vi "VelocityProfile.vi"(0 "t":dbl, 1 "a1":dbl=10.0, 3 "a3":dbl=15.0, 5 "s":dbl, 7 "intervalo":dbl=0.016, 9 "v_est":dbl, 11 "v_max":dbl=3.0, 12 "v3":dbl, 13 "s3":dbl) -> (4 "Velocity":dbl, 6 "VelocityProfileState Out":T1, 8 "Velocities":dbl[](array[numeric]), 10 "Time":dbl[](array[numeric]))   [LabVIEW 2023]
uses:
  Controle/VelocityProfileState.ctl
panel:
  out "Amax":dbl=8.0
  in  "Reset":bool
  out "Velocity Profile":cluster{dbl[], dbl[]}(graph)
  in  "Tolerancia Vel":dbl=0.01
  in  "Tolerancia Pos":dbl=0.010000000000000004
  out "VelocityProfileState In":T1={"t0"=0.0, "t1"=0.0, "t2"=0.0, "t3"=0.0, "v0"=0.0, "v_max"=3.0, "v3"=0.0, "v2"=0.0, "v1"=0.0, "perfil"=enum."Triangular", "regiao"=0, "s0"=0.0, "s1"=0.0, "s2"=0.0, "v"=0.0, "t"=0.0, "a1"=10.0, "s3"=0.0, "Reset"=FALSE, "s"=0.0, "a3"=15.0, "Ré"=FALSE, "Impossível"=FALSE, "intervalo"=0.0}
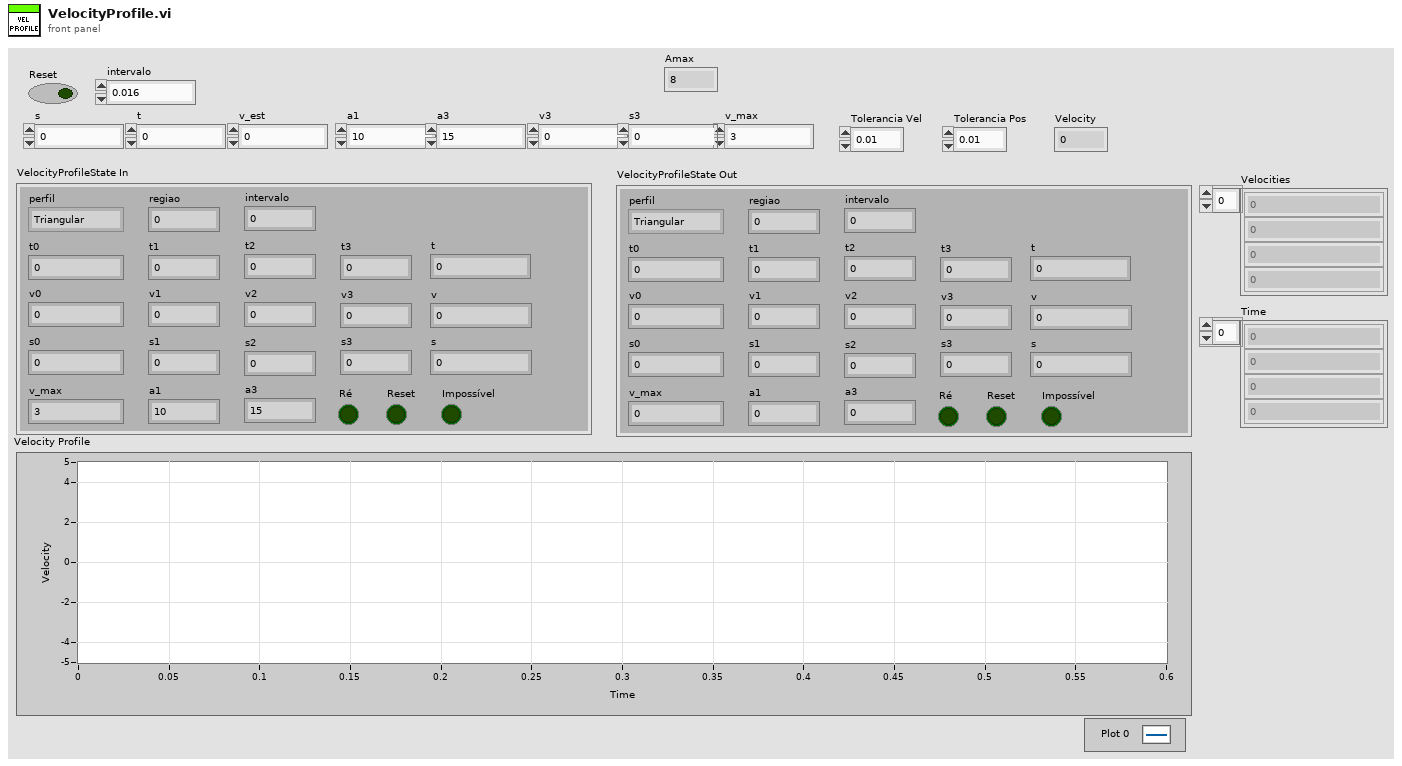
[diagram p1: front panel]
types:
  T1 = typedef "VelocityProfileState.ctl" = cluster{"t0":dbl, "t1":dbl, "t2":dbl, "t3":dbl, "v0":dbl, "v_max":dbl, "v3":dbl, "v2":dbl, "v1":dbl, "perfil":enum16{"Triangular", "Trapezoidal"}, "regiao":i32, "s0":dbl, "s1":dbl, "s2":dbl, "v":dbl, "t":dbl, "a1":dbl, "s3":dbl, "Reset":bool, "s":dbl, "a3":dbl, "Ré":bool, "Impossível":bool, "intervalo":dbl}
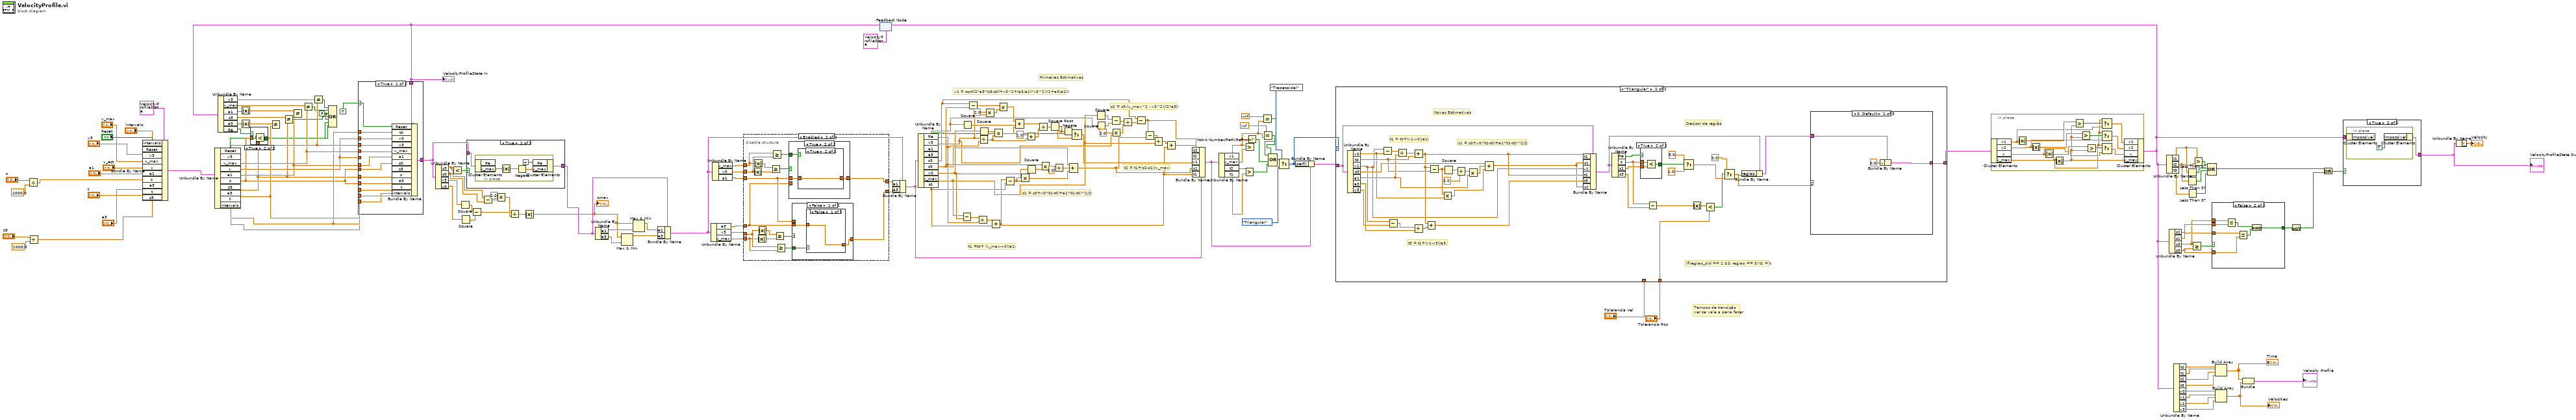
[diagram p0: block diagram]
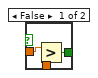
[diagram p2: hidden frame]
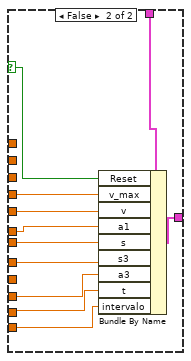
[diagram p3: hidden frame]
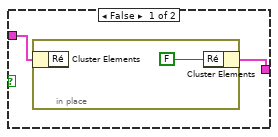
[diagram p4: hidden frame]
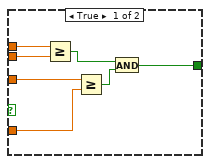
[diagram p5: hidden frame]
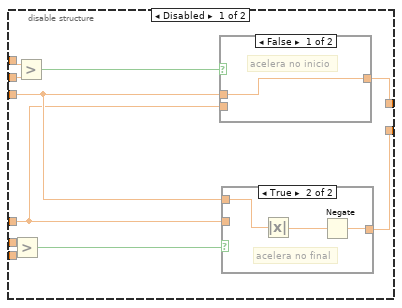
[diagram p6: hidden frame]
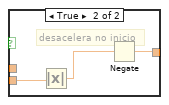
[diagram p8: hidden frame]
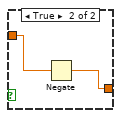
[diagram p9: hidden frame]
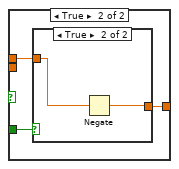
[diagram p10: hidden frame]
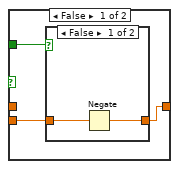
[diagram p12: hidden frame]
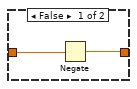
[diagram p14: hidden frame]
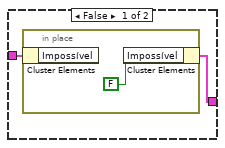
[diagram p15: hidden frame]
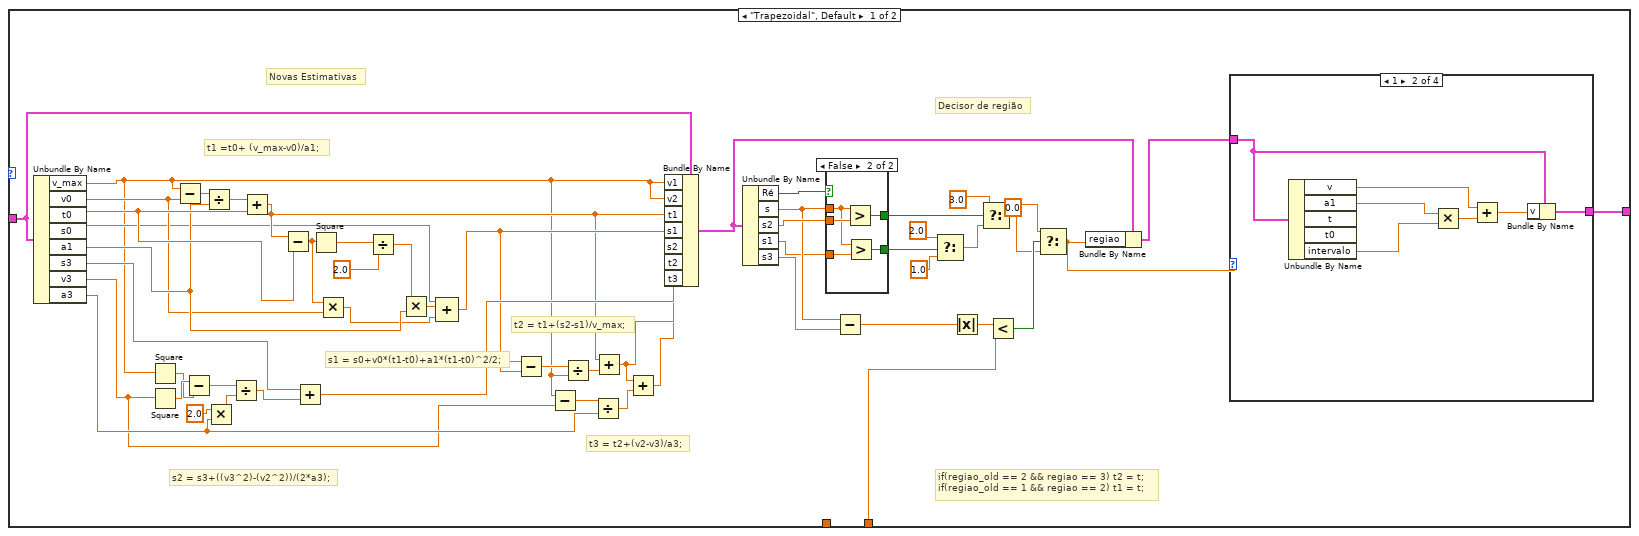
[diagram p16: hidden frame]
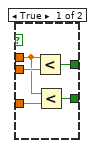
[diagram p17: hidden frame]
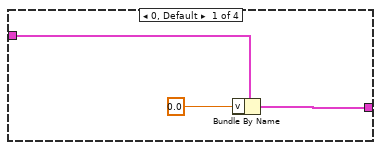
[diagram p18: hidden frame]
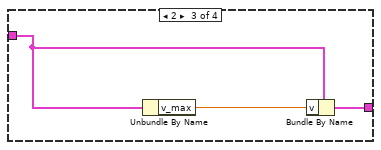
[diagram p19: hidden frame]
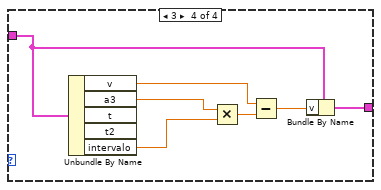
[diagram p20: hidden frame]
diagram:
  w40 = FALSE ("value")
  # "Tempos de transição\nver se vale a pena fazer"
  # "Primeiras Estimativas"
  # "t2 = t1+(s2-s1)/v_max;"
  # "s2 = s3-(v_max^2 - v3^2)/(2*a3);"
  # "s1 = s0+v0*(t1-t0)+a1*(t1-t0)^2/2;"
  # "t1 =t0+ (v_max-v0)/a1;"
  # "v1 = sqrt((2*a3*(s3-s0)+v3^2+(a3/a1)*v0^2)/(1+a3/a1));"
  n1 = Divide(x="s", y=1000.0) -> (x/y=w149:dbl)
  n2 = Divide(x="s3", y=1000.0) -> (x/y=w150:dbl)
  n3 = Bundle By Name(cluster=T1 {"t0"=0.0, "t1"=0.0, "t2"=0.0, "t3"=0.0, "v0"=0.0, "v_max"=0.0, "v3"=0.0, "v2"=0.0, "v1"=0.0, "perfil"=enum."Triangular", "regiao"=0, "s0"=0.0, "s1"=0.0, "s2"=0.0, "v"=0.0, "t"=0.0, "a1"=0.0, "s3"=0.0, "Reset"=FALSE, "s"=0.0, "a3"=0.0, "Ré"=FALSE, "Impossível"=FALSE, "intervalo"=0.0} ("VelocityProfileState In"), "intervalo"="intervalo", "Reset"="Reset", "v3"="v3", "v_max"="v_max", "v"="v_est", "a1"="a1", "s"=w149, "a3"="a3", "t"="t", "s3"=w150) -> (w155:T1)
  n4 = Unbundle By Name(w155) -> ("Reset"=w42:bool, "v3"=w128:dbl, "v_max"=w126:dbl, "v"=w56:dbl, "a1"=w55:dbl, "s"=w44:dbl, "s3"=w43:dbl, "a3"=w60:dbl, "t"=w57:dbl, "intervalo"=w35:dbl)
  n5 = feedback #1(T1 {"t0"=0.0, "t1"=0.0, "t2"=0.0, "t3"=0.0, "v0"=0.0, "v_max"=0.0, "v3"=0.0, "v2"=0.0, "v1"=0.0, "perfil"=enum."Triangular", "regiao"=0, "s0"=0.0, "s1"=0.0, "s2"=0.0, "v"=0.0, "t"=0.0, "a1"=0.0, "s3"=0.0, "Reset"=FALSE, "s"=0.0, "a3"=0.0, "Ré"=FALSE, "Impossível"=FALSE, "intervalo"=0.0} ("VelocityProfileState In")) -> (w25:T1)
  "VelocityProfileState In" <- w25
  n6 = Unbundle By Name(w25) -> ("v3"=w129:dbl, "v_max"=w127:dbl, "a1"=w48:dbl, "s3"=w125:dbl, "a3"=w47:dbl, "Ré"=w45:bool)
  n7 = Absolute Value(x=w48) -> (abs(x)=w49:dbl)
  n8 = Absolute Value(x=w47) -> (abs(x)=w46:dbl)
  n9 = case shown="True" w45 {
    tunnel: w44 -> [w167 w170]
    tunnel: w43 -> [w166 w169]
    tunnel: [w165 w168] -> w41
    frame False {
      n10 = Greater?(x=w167, y=w166) -> (0:w165:bool)
    }
    frame True {
      n11 = Less?(x=w170, y=w169) -> (x < y?=w168:bool)
    }
  }
  n12 = Not Equal?(x=w46, y=w60) -> ()  [unwired: 1 out]
  n13 = Not Equal?(x=w125, y=w43) -> (x != y?=w122:bool)
  n14 = Not Equal?(x=w49, y=w55) -> ()  [unwired: 1 out]
  n15 = Not Equal?(x=w127, y=w126) -> (x != y?=w123:bool)
  n16 = Not Equal?(x=w129, y=w128) -> (x != y?=w124:bool)
  n17 = Compound Arithmetic op=OR(w124, w123, w40, w122, w40, w41, w42) -> ()  [unwired: 1 out]
  n18 = case shown="True" TRUE {
    selector: TRUE -> [w178 w191]
    tunnel: w57 -> [w184 _]
    tunnel: w56 -> [w183 _]
    tunnel: w128 -> [w182 _]
    tunnel: w126 -> [w181 w195]
    tunnel: w56 -> [_ w194]
    tunnel: [w180 w193] -> w146
    tunnel: w25 -> [w179 w192]
    tunnel: w60 -> [w177 w190]
    tunnel: w57 -> [w176 w189]
    tunnel: w44 -> [w175 _]
    tunnel: w55 -> [w171 w188]
    tunnel: w44 -> [w174 w187]
    tunnel: w43 -> [w173 w186]
    tunnel: w35 -> [w172 w185]
    frame True {
      n19 = Bundle By Name(cluster=w179, "Reset"=w178, "t0"=w184, "v0"=w183, "v3"=w182, "v_max"=w181, "a1"=w171, "s0"=w174, "s3"=w173, "s"=w175, "a3"=w177, "t"=w176, "intervalo"=w172) -> (w180:T1)
    }
    frame False {
      n20 = Bundle By Name(cluster=w192, "Reset"=w191, "v_max"=w195, "v"=w194, "a1"=w188, "s"=w187, "s3"=w186, "a3"=w190, "t"=w189, "intervalo"=w185) -> (w193:T1)
    }
  }
  n21 = Unbundle By Name(w146) -> ("s3"=w10:dbl, "s0"=w9:dbl, "v3"=w14:dbl, "v0"=w13:dbl)
  n22 = Less?(x=w10, y=w9) -> (x < y?=w59:bool)
  n23 = Square(x=w14) -> (x^2=w12:dbl)
  n24 = Square(x=w13) -> (x^2=w11:dbl)
  n25 = case shown="True" w59 {
    tunnel: w146 -> [w197 w200]
    tunnel: [w196 w199] -> w21
    frame False {
      n26 = in-place {
        n27 = in-place-cluster #2(w197) -> ()  [unwired: 1 out]
        n28 = in-place-cluster #2("Ré"=FALSE) -> (w196:T1)
      }
    }
    frame True {
      n29 = in-place {
        n30 = in-place-cluster #3(w200) -> ("v_max"=w204:dbl)  [unwired: 1 out]
        n31 = Absolute Value(x=w204) -> (abs(x)=w203:dbl)
        n32 = Negate(x=w203) -> (-x=w202:dbl)
        n33 = in-place-cluster #3("Ré"=TRUE, "v_max"=w202) -> (w199:T1)
      }
    }
  }
  n34 = Subtract(x=w12, y=w11) -> (x-y=w6:dbl)
  n35 = Subtract(x=w10, y=w9) -> (x-y=w8:dbl)
  n36 = Multiply(x=2.0, y=w8) -> (x*y=w5:dbl)
  n37 = Divide(x=w6, y=w5) -> (x/y=w4:dbl)
  n38 = Absolute Value(x=w4) -> (abs(x)=w3:dbl)
  "Amax" <- w3
  n39 = Unbundle By Name(w21) -> ("a1"=w20:dbl, "a3"=w19:dbl)
  n40 = Max & Min(x=w3, y=w19) -> (max(x,y)=w1:dbl)  [unwired: 1 out]
  n41 = Max & Min(x=w3, y=w20) -> (max(x,y)=w2:dbl)  [unwired: 1 out]
  n42 = Bundle By Name(cluster=w21, "a1"=w2, "a3"=w1) -> (w22:T1)
  n43 = Unbundle By Name(w22) -> ("a3"=w61:dbl, "v3"=w106:dbl, "v_max"=w107:dbl)
  n44 = Unbundle By Name(w22) -> ("v_max"=w145:dbl, "v0"=w144:dbl, "a1"=w62:dbl)
  n45 = disable-structure shown="Enabled" {
    disable-tunnel: w145 -> [w214 w234]
    disable-tunnel: w144 -> [w213 w233]
    disable-tunnel: w107 -> [w212 w225]
    disable-tunnel: w106 -> [w211 w226]
    disable-tunnel: [w209 w232] -> w64
    disable-tunnel: [w207 w227] -> w63
    disable-tunnel: w62 -> [w206 w224]
    disable-tunnel: w61 -> [w205 w223]
    frame Disabled {
      n46 = Greater?(x=w211, y=w212) -> (0:w208:bool)
      n47 = Greater?(x=w214, y=w213) -> (0:w210:bool)
      n48 = case shown="False" w210 {
        tunnel: [w219 w221] -> w209
        tunnel: w206 -> [w219 _]
        tunnel: w205 -> [_ w222]
        frame False {
          # "acelera no inicio"
        }
        frame True {
          # "desacelera no inicio"
          n49 = Absolute Value(x=w222) -> (abs(x)=w220:dbl)
          n50 = Negate(x=w220) -> (-x=w221:dbl)
        }
      }
      n51 = case shown="True" w208 {
        tunnel: [w215 w218] -> w207
        tunnel: w206 -> [_ w216]
        tunnel: w205 -> [w215 _]
        frame False {
          # "desacelera no final"
        }
        frame True {
          # "acelera no final"
          n52 = Absolute Value(x=w216) -> (abs(x)=w217:dbl)
          n53 = Negate(x=w217) -> (-x=w218:dbl)
        }
      }
    }
    frame Enabled {
      n54 = Absolute Value(x=w233) -> (abs(x)=w237:dbl)
      n55 = Absolute Value(x=w234) -> (abs(x)=w238:dbl)
      n56 = Absolute Value(x=w225) -> (abs(x)=w229:dbl)
      n57 = Absolute Value(x=w226) -> (abs(x)=w228:dbl)
      n58 = Greater Or Equal?(x=w238, y=w237) -> (x >= y?=w236:bool)
      n59 = Greater Or Equal?(x=w234, y=w233) -> (x >= y?=w235:bool)
      n60 = Greater Or Equal?(x=w228, y=w229) -> (x >= y?=w230:bool)
      n61 = Greater Or Equal?(x=w226, y=w225) -> (x >= y?=w231:bool)
      n62 = case shown="True" w236 {
        tunnel: w224 -> [_ w257]
        tunnel: w235 -> [w253 w259]
        tunnel: [w252 w258] -> w232
        tunnel: w223 -> [w251 _]
        frame False {
          n63 = case shown="False" w253 {
            tunnel: [w254 w256] -> w252
            tunnel: w251 -> [w255 w256]
            frame False {
              n64 = Negate(x=w255) -> (-x=w254:dbl)
            }
            frame True {
            }
          }
        }
        frame True {
          n65 = case shown="True" w259 {
            tunnel: [w260 w262] -> w258
            tunnel: w257 -> [w261 w262]
            frame False {
              n66 = Negate(x=w261) -> (-x=w260:dbl)
            }
            frame True {
            }
          }
        }
      }
      n67 = case shown="False" w230 {
        tunnel: w231 -> [w241 w247]
        tunnel: [w240 w246] -> w227
        tunnel: w224 -> [_ w245]
        tunnel: w223 -> [w239 _]
        frame False {
          n68 = case shown="False" w241 {
            tunnel: [w242 w243] -> w240
            tunnel: w239 -> [w242 w244]
            frame False {
            }
            frame True {
              n69 = Negate(x=w244) -> (-x=w243:dbl)
            }
          }
        }
        frame True {
          n70 = case shown="True" w247 {
            tunnel: [w248 w250] -> w246
            tunnel: w245 -> [w248 w249]
            frame False {
            }
            frame True {
              n71 = Negate(x=w249) -> (-x=w250:dbl)
            }
          }
        }
      }
    }
  }
  n72 = Bundle By Name(cluster=w22, "a1"=w64, "a3"=w63) -> (w65:T1)
  n73 = Unbundle By Name(w65) -> ("Ré"=w58:bool, "v3"=w80:dbl, "a1"=w98:dbl, "a3"=w77:dbl, "s3"=w74:dbl, "s0"=w97:dbl, "v0"=w96:dbl, "v_max"=w72:dbl, "t0"=w105:dbl)
  n74 = Subtract(x=w72, y=w96) -> (x-y=w143:dbl)
  n75 = Square(x=w80) -> (x^2=w93:dbl)
  n76 = Subtract(x=w74, y=w97) -> (x-y=w92:dbl)
  n77 = Divide(x=w143, y=w98) -> (x/y=w142:dbl)
  n78 = Divide(x=w77, y=w98) -> (x/y=w86:dbl)
  n79 = Square(x=w96) -> (x^2=w95:dbl)
  n80 = Multiply(x=2.0, y=w77) -> (x*y=w91:dbl)
  n81 = Add(x=w142, y=w105) -> (x+y=w70:dbl)
  n82 = Multiply(x=w95, y=w86) -> (x*y=w94:dbl)
  n83 = Multiply(x=w92, y=w91) -> (x*y=w89:dbl)
  n84 = Subtract(x=w70, y=w105) -> (x-y=w104:dbl)
  n85 = Compound Arithmetic op=ADD(w89, w93, w94) -> (w88:dbl)
  n86 = Multiply(x=w96, y=w104) -> (x*y=w99:dbl)
  n87 = Add(x=1.0, y=w86) -> (x+y=w87:dbl)
  n88 = Square(x=w104) -> (x^2=w103:dbl)
  n89 = Divide(x=w88, y=w87) -> (x/y=w84:dbl)
  n90 = Multiply(x=w98, y=w103) -> (x*y=w102:dbl)
  n91 = Square Root(x=w84) -> (sqrt(x)=w83:dbl)
  n92 = Divide(x=w102, y=2.0) -> (x/y=w100:dbl)
  n93 = Negate(x=w83) -> (-x=w110:dbl)
  n94 = Compound Arithmetic op=ADD(w97, w100, w99) -> (w66:dbl)
  n95 = Select(t=w110, s=w58, f=w83) -> (s? t:f=w67:dbl)
  n96 = Square(x=w72) -> (x^2=w82:dbl)
  n97 = Square(x=w80) -> (x^2=w81:dbl)
  n98 = Subtract(x=w82, y=w81) -> (x-y=w79:dbl)
  n99 = Multiply(x=2.0, y=w77) -> (x*y=w78:dbl)
  n100 = Divide(x=w79, y=w78) -> (x/y=w75:dbl)
  n101 = Subtract(x=w74, y=w75) -> (x-y=w69:dbl)
  n102 = Subtract(x=w69, y=w66) -> (x-y=w73:dbl)
  n103 = Divide(x=w73, y=w72) -> (x/y=w71:dbl)
  n104 = Add(x=w71, y=w70) -> (x+y=w68:dbl)
  n105 = Bundle By Name(cluster=w65, "s2"=w69, "t2"=w68, "v1"=w67, "s1"=w66, "t1"=w70) -> (w134:T1)
  n106 = Unbundle By Name(w134) -> ("v1"=w18:dbl, "v_max"=w141:dbl, "t2"=w140:dbl, "t1"=w139:dbl)
  n107 = Greater?(x=w140, y=w139) -> (0:w39:bool)
  n108 = Greater?(x=w18, y=w141) -> ()  [unwired: 1 out]
  n109 = Not A Number/Path/Refnum?(number/path/refnum=w18) -> (NaN/Path/Refnum?=w108:bool)
  n110 = Equal?(x=-inf, y=w18) -> (x = y?=w16:bool)
  n111 = Equal?(x=inf, y=w18) -> (x = y?=w38:bool)
  n112 = Compound Arithmetic op=OR(w16, w38, w108, w39) -> (w109:bool)
  n113 = Select(t=enum16{"Triangular", "Trapezoidal"}."Trapezoidal" ("perfil"), s=w109, f=enum16{"Triangular", "Trapezoidal"}."Triangular" ("perfil")) -> (s? t:f=w136:enum16{"Triangular", "Trapezoidal"})
  n114 = Bundle By Name(cluster=w134, "perfil"=w136) -> (w135:T1)
  n115 = case shown="\"Triangular\"" w136 {
    tunnel: w135 -> [w315 w375]
    tunnel: [w303 w362] -> w131
    tunnel: "Tolerancia Pos" -> [w286 w360]
    tunnel: "Tolerancia Vel" -> [_ _]
    frame "Trapezoidal", Default {
      # "t3 = t2+(v2-v3)/a3;"
      # "t2 = t1+(s2-s1)/v_max;"
      # "s2 = s3+((v3^2)-(v2^2))/(2*a3);"
      # "s1 = s0+v0*(t1-t0)+a1*(t1-t0)^2/2;"
      # "t1 =t0+ (v_max-v0)/a1;"
      # "if(regiao_old == 2 && regiao == 3) t2 = t;\nif(regiao_old == 1 && regiao == 2) t1 = t;"
      # "Decisor de região"
      # "Novas Estimativas"
      n116 = Unbundle By Name(w315) -> ("v_max"=w268:dbl, "v0"=w280:dbl, "t0"=w290:dbl, "s0"=w279:dbl, "a1"=w289:dbl, "s3"=w270:dbl, "v3"=w266:dbl, "a3"=w273:dbl)
      n117 = Square(x=w268) -> (x^2=w276:dbl)
      n118 = Square(x=w266) -> (x^2=w277:dbl)
      n119 = Subtract(x=w268, y=w280) -> (x-y=w302:dbl)
      n120 = Subtract(x=w277, y=w276) -> (x-y=w275:dbl)
      n121 = Divide(x=w302, y=w289) -> (x/y=w301:dbl)
      n122 = Multiply(x=2.0, y=w273) -> (x*y=w274:dbl)
      n123 = Divide(x=w275, y=w274) -> (x/y=w271:dbl)
      n124 = Add(x=w301, y=w290) -> (x+y=w293:dbl)
      n125 = Subtract(x=w293, y=w290) -> (x-y=w281:dbl)
      n126 = Add(x=w270, y=w271) -> (x+y=w296:dbl)
      n127 = Square(x=w281) -> (x^2=w300:dbl)
      n128 = Multiply(x=w281, y=w280) -> (x*y=w278:dbl)
      n129 = Divide(x=w300, y=2.0) -> (x/y=w298:dbl)
      n130 = Multiply(x=w298, y=w289) -> (x*y=w297:dbl)
      n131 = Compound Arithmetic op=ADD(w279, w297, w278) -> (w295:dbl)
      n132 = Subtract(x=w296, y=w295) -> (x-y=w269:dbl)
      n133 = Subtract(x=w268, y=w266) -> (x-y=w267:dbl)
      n134 = Divide(x=w269, y=w268) -> (x/y=w294:dbl)
      n135 = Divide(x=w267, y=w273) -> (x/y=w291:dbl)
      n136 = Add(x=w293, y=w294) -> (x+y=w292:dbl)
      n137 = Add(x=w292, y=w291) -> (x+y=w288:dbl)
      n138 = Bundle By Name(cluster=w315, "v1"=w268, "v2"=w268, "t1"=w293, "s1"=w295, "s2"=w296, "t2"=w292, "t3"=w288) -> (w306:T1)
      n139 = Unbundle By Name(w306) -> ("Ré"=w265:bool, "s"=w311:dbl, "s2"=w314:dbl, "s1"=w264:dbl, "s3"=w285:dbl)
      n140 = case shown="False" w265 {
        tunnel: w314 -> [w320 w325]
        tunnel: [w319 w324] -> w313
        tunnel: w311 -> [w318 w323]
        tunnel: w264 -> [w317 w322]
        tunnel: [w316 w321] -> w263
        frame True {
          n141 = Less?(x=w318, y=w320) -> (x < y?=w319:bool)
          n142 = Less?(x=w318, y=w317) -> (x < y?=w316:bool)
        }
        frame False {
          n143 = Greater?(x=w323, y=w325) -> (0:w324:bool)
          n144 = Greater?(x=w323, y=w322) -> (0:w321:bool)
        }
      }
      n145 = Subtract(x=w311, y=w285) -> (x-y=w310:dbl)
      n146 = Select(t=2.0, s=w263, f=1.0) -> (s? t:f=w282:dbl)
      n147 = Absolute Value(x=w310) -> (abs(x)=w309:dbl)
      n148 = Select(t=3.0, s=w313, f=w282) -> (s? t:f=w287:dbl)
      n149 = Less?(x=w309, y=w286) -> (x < y?=w308:bool)
      n150 = Select(t=0.0, s=w308, f=w287) -> (s? t:f=w305:dbl)
      n151 = Bundle By Name(cluster=w306, "regiao"=w305) -> (w304:T1)
      n152 = case shown="1" w305 {
        tunnel: w304 -> [w328 w335 w337 w345]
        tunnel: [w326 w334 w338 w344] -> w303
        frame 0, Default {
          n153 = Bundle By Name(cluster=w328, "v"=0.0) -> (w326:T1)
        }
        frame 1 {
          n154 = Unbundle By Name(w335) -> ("v"=w331:dbl, "a1"=w333:dbl, "intervalo"=w329:dbl)  [unwired: 2 out]
          n155 = Multiply(x=w333, y=w329) -> (x*y=w332:dbl)
          n156 = Add(x=w331, y=w332) -> (x+y=w330:dbl)
          n157 = Bundle By Name(cluster=w335, "v"=w330) -> (w334:T1)
        }
        frame 2 {
          n158 = Unbundle By Name(w337) -> ("v_max"=w336:dbl)
          n159 = Bundle By Name(cluster=w337, "v"=w336) -> (w338:T1)
        }
        frame 3 {
          n160 = Unbundle By Name(w345) -> ("v"=w341:dbl, "a3"=w343:dbl, "intervalo"=w339:dbl)  [unwired: 2 out]
          n161 = Multiply(x=w343, y=w339) -> (x*y=w342:dbl)
          n162 = Subtract(x=w341, y=w342) -> (x-y=w340:dbl)
          n163 = Bundle By Name(cluster=w345, "v"=w340) -> (w344:T1)
        }
      }
    }
    frame "Triangular" {
      # "if(regiao_old == 1 && regiao == 3) t1 = t;"
      # "Decisor de região"
      # "Novas Estimativas"
      # "t3 = t1+(v1-v3)/a3;"
      # "s1 = s0+v0*(t1-t0)+a1*(t1-t0)^2/2;"
      # "t1 = t0+(v1-v0)/a1;"
      n164 = Unbundle By Name(w375) -> ("v0"=w348:dbl, "t0"=w381:dbl, "v1"=w352:dbl, "s0"=w378:dbl, "a1"=w355:dbl, "a3"=w354:dbl, "v3"=w351:dbl)
      n165 = Subtract(x=w352, y=w348) -> (x-y=w383:dbl)
      n166 = Subtract(x=w352, y=w351) -> (x-y=w353:dbl)
      n167 = Divide(x=w383, y=w355) -> (x/y=w382:dbl)
      n168 = Add(x=w382, y=w381) -> (x+y=w376:dbl)
      n169 = Divide(x=w353, y=w354) -> (x/y=w377:dbl)
      n170 = Add(x=w376, y=w377) -> (x+y=w350:dbl)
      n171 = Subtract(x=w376, y=w381) -> (x-y=w349:dbl)
      n172 = Multiply(x=w349, y=w348) -> (x*y=w347:dbl)
      n173 = Square(x=w349) -> (x^2=w380:dbl)
      n174 = Divide(x=w380, y=2.0) -> (x/y=w357:dbl)
      n175 = Multiply(x=w357, y=w355) -> (x*y=w356:dbl)
      n176 = Compound Arithmetic op=ADD(w378, w356, w347) -> (w361:dbl)
      n177 = Bundle By Name(cluster=w375, "t1"=w376, "s1"=w361, "v2"=w352, "t2"=w376, "t3"=w350, "s2"=w361) -> (w365:T1)
      n178 = Unbundle By Name(w365) -> ("Ré"=w346:bool, "s"=w371:dbl, "s1"=w374:dbl, "s3"=w370:dbl)
      n179 = case shown="True" w346 {
        tunnel: w374 -> [w386 w387]
        tunnel: [w385 w389] -> w373
        tunnel: w371 -> [w384 w388]
        frame False {
          n180 = Greater?(x=w384, y=w386) -> (0:w385:bool)
        }
        frame True {
          n181 = Less?(x=w388, y=w387) -> (x < y?=w389:bool)
        }
      }
      n182 = Subtract(x=w371, y=w370) -> (x-y=w369:dbl)
      n183 = Select(t=3.0, s=w373, f=1.0) -> (s? t:f=w367:dbl)
      n184 = Absolute Value(x=w369) -> (abs(x)=w368:dbl)
      n185 = Less?(x=w368, y=w360) -> (x < y?=w366:bool)
      n186 = Select(t=0.0, s=w366, f=w367) -> (s? t:f=w364:dbl)
      n187 = Bundle By Name(cluster=w365, "regiao"=w364) -> (w363:T1)
      n188 = case shown="0, Default" w364 {
        tunnel: w363 -> [w392 w399 w406]
        tunnel: [w390 w398 w405] -> w362
        frame 0, Default {
          n189 = Bundle By Name(cluster=w392, "v"=0.0) -> (w390:T1)
        }
        frame 1 {
          n190 = Unbundle By Name(w399) -> ("v"=w395:dbl, "a1"=w397:dbl, "intervalo"=w393:dbl)  [unwired: 2 out]
          n191 = Multiply(x=w397, y=w393) -> (x*y=w396:dbl)
          n192 = Add(x=w395, y=w396) -> (x+y=w394:dbl)
          n193 = Bundle By Name(cluster=w399, "v"=w394) -> (w398:T1)
        }
        frame 3 {
          n194 = Unbundle By Name(w406) -> ("v"=w402:dbl, "a3"=w404:dbl, "intervalo"=w400:dbl)  [unwired: 2 out]
          n195 = Multiply(x=w404, y=w400) -> (x*y=w403:dbl)
          n196 = Subtract(x=w402, y=w403) -> (x-y=w401:dbl)
          n197 = Bundle By Name(cluster=w406, "v"=w401) -> (w405:T1)
        }
      }
    }
  }
  n198 = in-place {
    n199 = in-place-cluster #4(w131) -> ("v1"=w409:dbl, "v2"=w408:dbl, "v"=w407:dbl, "v_max"=w410:dbl)
    n200 = Absolute Value(x=w409) -> (abs(x)=w415:dbl)
    n201 = Absolute Value(x=w408) -> (abs(x)=w414:dbl)
    n202 = Absolute Value(x=w407) -> (abs(x)=w413:dbl)
    n203 = Absolute Value(x=w410) -> (abs(x)=w412:dbl)
    n204 = Greater?(x=w415, y=w412) -> (0:w420:bool)
    n205 = Greater?(x=w414, y=w412) -> (0:w419:bool)
    n206 = Greater?(x=w413, y=w412) -> (0:w411:bool)
    n207 = Select(t=w410, s=w420, f=w409) -> (s? t:f=w418:dbl)
    n208 = Select(t=w410, s=w419, f=w408) -> (s? t:f=w417:dbl)
    n209 = Select(t=w410, s=w411, f=w407) -> (s? t:f=w416:dbl)
    n210 = in-place-cluster #4("v1"=w418, "v2"=w417, "v"=w416, "v_max"=w412) -> (w34:T1)
  }
  n211 = feedback-in #1(w34) -> ()
  n212 = Unbundle By Name(w34) -> ("t1"=w54:dbl, "t2"=w24:dbl, "t3"=w51:dbl)
  n213 = Unbundle By Name(w34) -> ("s2"=w30:dbl, "s1"=w32:dbl, "s3"=w29:dbl, "s0"=w31:dbl)
  n214 = Unbundle By Name(w34) -> ("t0"=w120:dbl, "t1"=w119:dbl, "t2"=w118:dbl, "t3"=w117:dbl, "v0"=w116:dbl, "v1"=w115:dbl, "v2"=w114:dbl, "v3"=w113:dbl)
  n215 = Less Than 0?(x=w54) -> (x < 0?=w53:bool)
  n216 = Less Than 0?(x=w24) -> (x < 0?=w52:bool)
  n217 = Less Than 0?(x=w51) -> (x < 0?=w50:bool)
  n218 = Greater Or Equal?(x=w29, y=w31) -> (x >= y?=w33:bool)
  n219 = Greater?(x=w54, y=w24) -> (0:w23:bool)
  n220 = Compound Arithmetic op=OR(w23, w53, w52, w50) -> (w28:bool)
  n221 = case shown="False" w33 {
    tunnel: w32 -> [w426 w433]
    tunnel: w31 -> [w427 w434]
    tunnel: w30 -> [w425 w432]
    tunnel: w29 -> [w424 w431]
    tunnel: [w421 w428] -> w27
    frame True {
      n222 = Greater Or Equal?(x=w424, y=w425) -> (x >= y?=w422:bool)
      n223 = Greater Or Equal?(x=w426, y=w427) -> (x >= y?=w423:bool)
      n224 = And(x=w422, y=w423) -> (x .and. y?=w421:bool)
    }
    frame False {
      n225 = Less Or Equal?(x=w431, y=w432) -> (x <= y?=w429:bool)
      n226 = Less Or Equal?(x=w433, y=w434) -> (x <= y?=w430:bool)
      n227 = And(x=w429, y=w430) -> (x .and. y?=w428:bool)
    }
  }
  n228 = Build Array(w120, w119, w118, w117) -> (w112:dbl[])
  "Time" <- w112
  n229 = Build Array(w116, w115, w114, w113) -> (w111:dbl[])
  "Velocities" <- w111
  n230 = Bundle(w112, w111) -> (→"Velocity Profile":cluster{dbl[], dbl[]})  [unwired: 1 in]
  n231 = Not(x=w27) -> (.not. x?=w26:bool)
  n232 = Or(x=w28, y=w26) -> (x .or. y?=w15:bool)
  n233 = case shown="True" w15 {
    tunnel: w34 -> [w436 w439]
    tunnel: [w435 w438] -> w161
    frame False {
      n234 = in-place {
        n235 = in-place-cluster #5(w436) -> ()  [unwired: 1 out]
        n236 = in-place-cluster #5("Impossível"=FALSE) -> (w435:T1)
      }
    }
    frame True {
      n237 = in-place {
        n238 = in-place-cluster #6(w439) -> ()  [unwired: 1 out]
        n239 = in-place-cluster #6("Impossível"=TRUE) -> (w438:T1)
      }
    }
  }
  "VelocityProfileState Out" <- w161
  n240 = Unbundle By Name(w161) -> ("v"=→"Velocity":dbl)
